vi "Build diode path.vi"(0 "Data dir":path) -> (7 "Diode write path":path, 10 "error out":errorcluster)   [LabVIEW 2018]
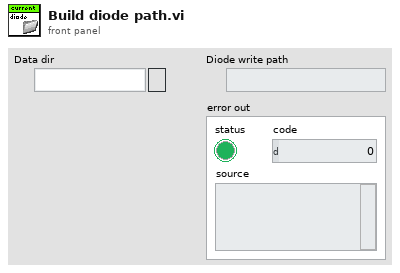
[diagram p1: front panel]
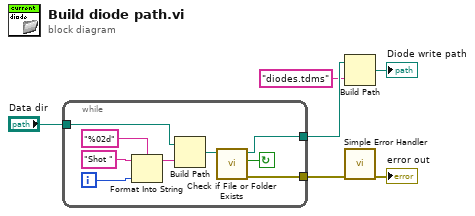
[diagram p0: block diagram]
diagram:
  n1 = while {
    tunnel: "Data dir" -> [w13]
    tunnel: [w9] -> w5
    tunnel: [w7] -> w1
    i -> [w10]
    stop <- w8 continue-if-true
    n2 = Format Into String(format string="%02d", initial string="Shot ", w10) -> (resulting string=w12:string)  [unwired: 1 in, 1 out]
    n3 = Build Path(base path=w13, name or relative path=w12) -> (appended path=w11:path)
    n4 = call <vilib>:"Check if File or Folder Exists.vi"("path"=w11) -> ("error out"=w7:errorcluster, "file or folder exists?"=w8:bool, "dup path"=w9:path)  [unwired: 8 in]
  }
  n5 = Build Path(base path=w5, name or relative path="diodes.tdms") -> (appended path=→"Diode write path":path)
  n6 = call <vilib>:"Simple Error Handler.vi"("error in (no error)"=w1) -> ("error out"=→"error out":errorcluster)  [unwired: 4 in, 4 out]
